vi "Test-Elevator.vi"() -> ()   [LabVIEW 2023]
doc: "This VI implements the framework and scheduler for your robotics program. It should not be necessary to modify the framework. You are expected to add your code to the VIs called from Robot Main - the ones located in the Team Code folder within the project."
uses:
  <vilib>/Rock Robotics/WPI/DriverStation/WPI_DriverStationRobotMode2.ctl
  Robot Global Data.vi
  Elevator/ElevatorL4SendCmd.vi
  Elevator/ElevatorAlgae1SendCmd.vi
  Elevator/ElevatorL3SendCmd.vi
  Elevator/ElevatorAlgae2SendCmd.vi
  Elevator/ElevatorSourceSendCmd.vi
  Elevator/ElevatorL2SendCmd.vi
  Elevator/ElevatorRestSendCmd.vi
  Elevator/ElevatorL1SendCmd.vi
  Elevator/ElevatorGlobal.vi
  <vilib>/Rock Robotics/WPI/ThirdParty/JAS_Junk/TrajLib/Trajectory_Library.lvlib
panel:
  out "Battery_Volts":dbl format="%9.1f"
  out "L4 2":bool
  out "HeightSP_Inch":dbl format="%9.1f"
  in  "Rest":bool
  out "HighLimitSwitch":bool
  in  "CmdSpecific":bool
  in  "Specific":dbl
  in  "Algae2":bool
  in  "L4":bool
  in  "Source":bool
  out "Low Limit Switch":bool
  out "HeightInch":dbl format="%9.1f"
  in  "L1":bool
  in  "L2":bool
  in  "Algae1":bool
  in  "L3":bool
  out "Robot Mode":T1
  out "MotorOutDmd":dbl format="%9.2f"
  in  "error in (no error)":errorcluster
  in  "Finish":bool
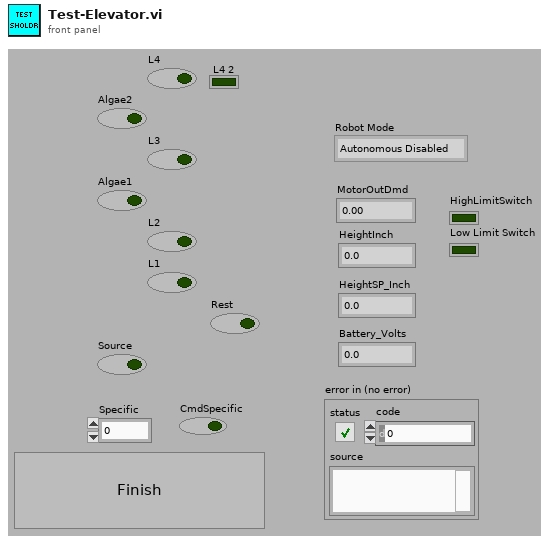
[diagram p1: front panel]
types:
  T1 = typedef "WPI_DriverStationRobotMode2.ctl" = enum16{"Autonomous Disabled", "Autonomous Enabled", "Teleop Disabled", "Teleop Enabled", "Disconnected", "Finish", "Test Disabled", "Test Enabled", "Emergency Stopped"}
  T2 = typedef "WPI_DriverStationMatch Info.ctl" = cluster{"Autonomous Elapsed Seconds":dbl, "TeleOp Elapsed Seconds":dbl, "Disabled Elapsed Seconds":dbl, "Visited Autonomous":bool, "Visited TeleOp":bool, "Visited Disabled":bool, "Autonomous Settings":cluster{"Autonomous Style":enum16{"Iterative", "Independent"}, "VI Refnum":refnum<vi>}}
  T3 = typedef "WPI_DriverStationDerivedRobotMode.ctl" = enum16{"Init", "Execute", "Stop"}
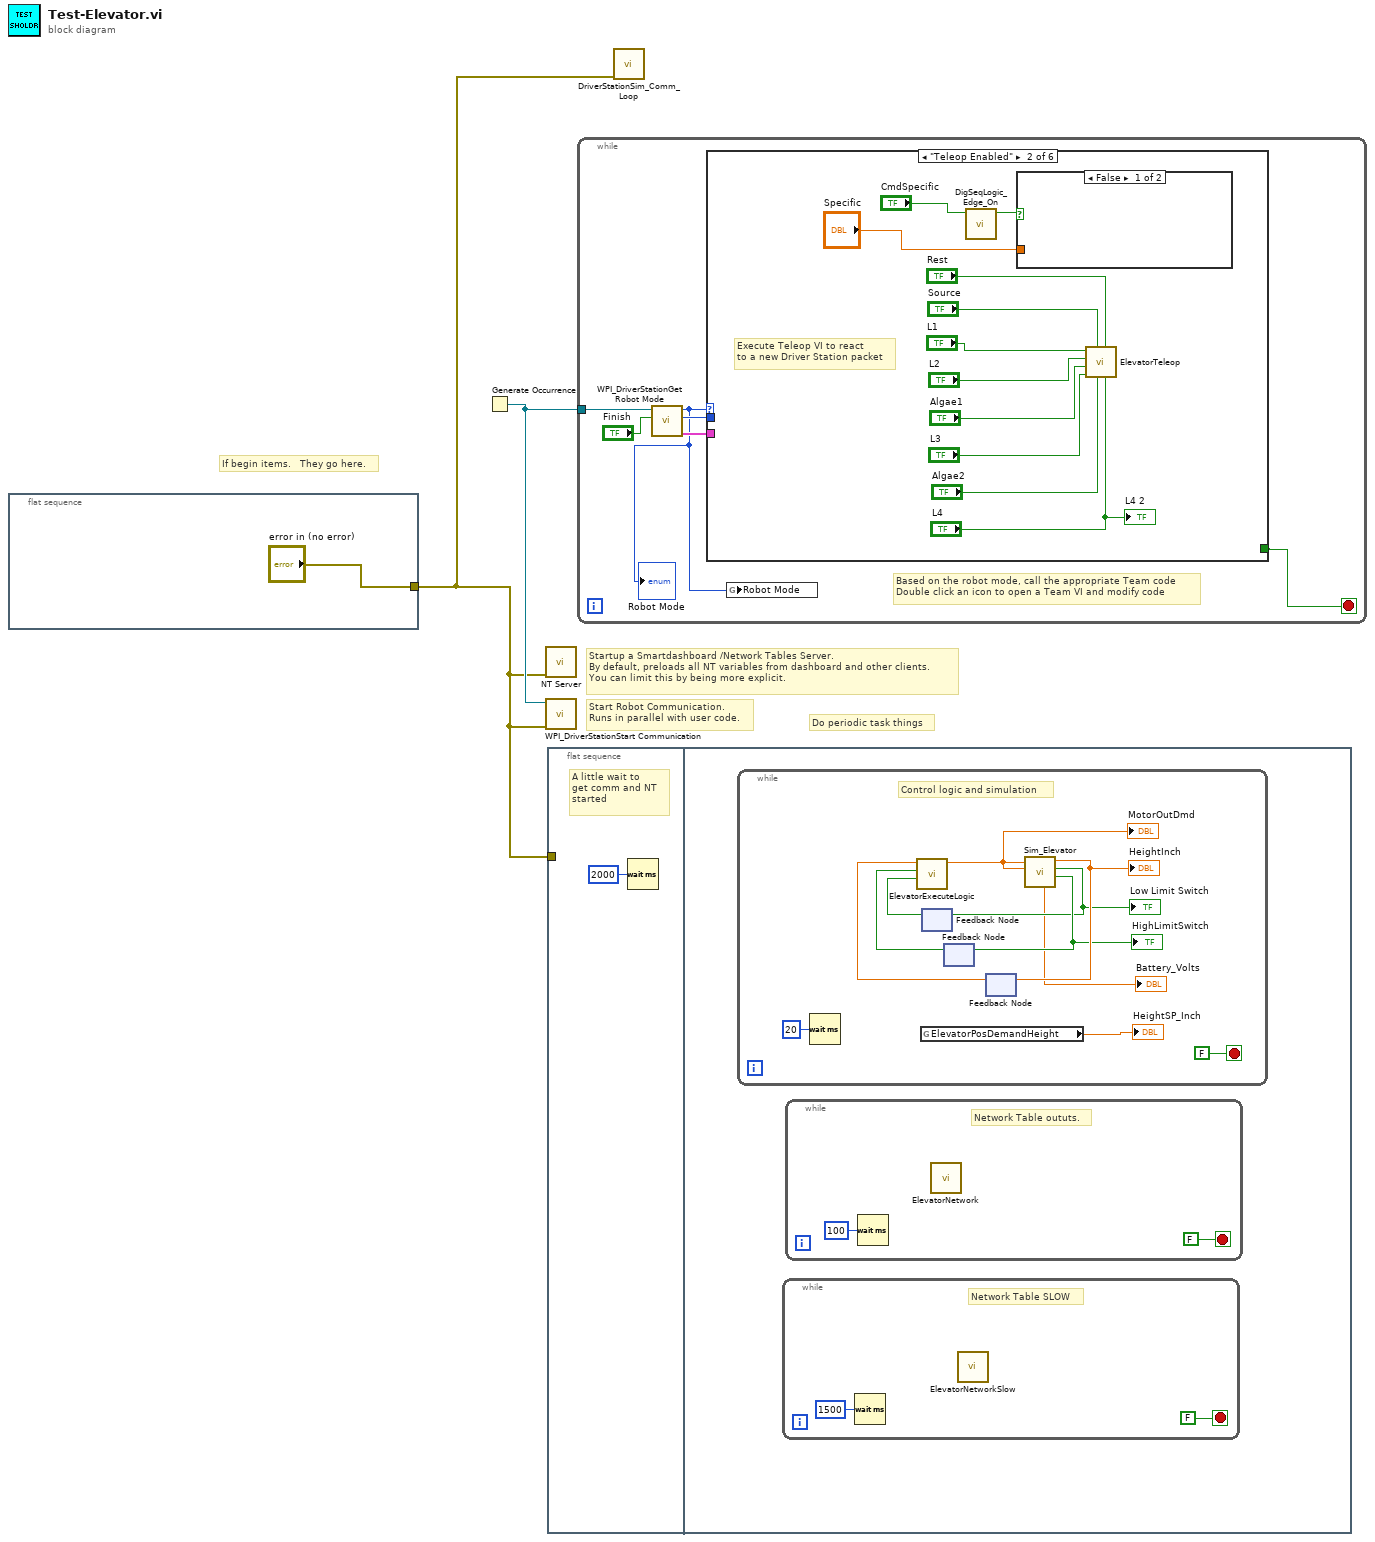
[diagram p0: block diagram]
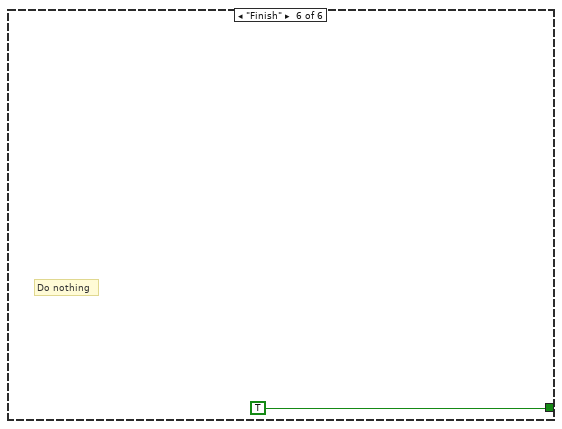
[diagram p7: hidden frame]
diagram:
  # "If begin items.   They go here."
  # "Do periodic task things"
  # "Startup a Smartdashboard /Network Tables Server.\nBy default, preloads all NT variables from dashboard and other clients.\nYou can limit this by being more explicit."
  # "Start Robot Communication.\nRuns in parallel with user code."
  n1 = flat-sequence {
    tunnel: ["error in (no error)"] -> w1
    frame #0 {
    }
  }
  n2 = Generate Occurrence() -> (w2:refnum<k4>)
  n3 = call <vilib>:"NT Server.vi"("error in (no error)"=w1) -> ()  [unwired: 10 in, 1 out]
  n4 = call <vilib>:"WPI_DriverStationStart Communication.vi"("error in (no error)"=w1, "occurrence"=w2) -> ()  [unwired: 1 in, 9 out]
  n5 = flat-sequence {
    tunnel: w1 -> [_]
    frame #0 {
      # "A little wait to\nget comm and NT\nstarted"
      n6 = Wait (ms)(milliseconds to wait=u32 2000) -> ()  [unwired: 1 out]
    }
    frame #1 {
      n7 = while {
        stop <- FALSE stop-if-true
        # "Control logic and simulation"
        n8 = Wait (ms)(milliseconds to wait=u32 20) -> ()  [unwired: 1 out]
        n9 = global read "ElevatorGlobal.vi" "ElevatorPosDemandHeight"() -> (→"HeightSP_Inch":dbl)
        n10 = feedback #1() -> (w13:bool)  [unwired: 1 in]
        n11 = feedback #2() -> (w15:bool)  [unwired: 1 in]
        n12 = feedback #3() -> (w17:dbl)  [unwired: 1 in]
        n13 = call "ElevatorExecuteLogic.vi"("LowLimitSwitch"=w13, "HighLimitSwitch"=w15, "PositionHeight"=w17) -> ("MotorDemand"=w12:dbl)  [unwired: 7 in, 1 out]
        "MotorOutDmd" <- w12
        n14 = call "Sim_Elevator.vi"("Motor2 Dmd"=w12, "Motor1 Dmd"=w12) -> ("HighLimitSwitch"=w16:bool, "Low Limit Switch"=w14:bool, "ElevHeightInch"=w18:dbl, "Voltage"=→"Battery_Volts":dbl)  [unwired: 6 in]
        "HeightInch" <- w18
        "Low Limit Switch" <- w14
        "HighLimitSwitch" <- w16
        n15 = feedback-in #1(w14) -> ()
        n16 = feedback-in #2(w16) -> ()
        n17 = feedback-in #3(w18) -> ()
      }
      n18 = while {
        stop <- FALSE stop-if-true
        # "Network Table SLOW"
        n19 = Wait (ms)(milliseconds to wait=u32 1500) -> ()  [unwired: 1 out]
        n20 = call "ElevatorNetworkSlow.vi"() -> ()  [unwired: 11 in, 1 out]
      }
      n21 = while {
        stop <- FALSE stop-if-true
        # "Network Table oututs."
        n22 = Wait (ms)(milliseconds to wait=u32 100) -> ()  [unwired: 1 out]
        n23 = call "ElevatorNetwork.vi"() -> ()  [unwired: 11 in, 1 out]
      }
    }
  }
  n24 = while {
    tunnel: w2 -> [w25]
    stop <- w20 stop-if-true
    # "Based on the robot mode, call the appropriate Team code\nDouble click an icon to open a Team VI and modify code"
    n25 = call <vilib>:"WPI_DriverStationGet Robot Mode.vi"("Finish"="Finish", "DS Occurrence"=w25) -> ("Match Info out"=w22:T2, "Call Context"=w24:T3, "Robot Mode"=w21:T1)  [unwired: 7 out]
    "Robot Mode" <- w21
    n26 = case shown="\"Teleop Enabled\"" w21 {
      tunnel: w24 -> [_ _ _ _ _ _]
      tunnel: w22 -> [_ _ _ _ _ _]
      tunnel: [_ _ _ _ _ TRUE] -> w20
      frame "Autonomous Enabled" {
        # "Do nothing...."
      }
      frame "Teleop Enabled" {
        # "Execute Teleop VI to react\nto a new Driver Station packet"
        n27 = call <vilib>:"DigSeqLogic_Edge_On.vi"("Input"="CmdSpecific") -> ("On Edge"=w36:bool)  [unwired: 10 in]
        n28 = case shown="False" w36 {
          tunnel: "Specific" -> [_ _]
          frame False {
          }
          frame True {
          }
        }
        n29 = call "ElevatorTeleop.vi"("CmdElevL4"="L4", "CmdElevRest"="Rest", "CmdElevAlgae2"="Algae2", "CmdElevSource"="Source", "CmdElevL3"="L3", "CmdElevAlgae1"="Algae1", "CmdElevL2"="L2", "CmdElevL1"="L1") -> ()  [unwired: 4 in]
        "L4 2" <- "L4"
      }
      frame "Test Disabled", "Test Enabled" {
        # "Do nothing"
      }
      frame "Autonomous Disabled", "Teleop Disabled" {
        # "Do nothing."
      }
      frame "Disconnected", Default {
        # "Driver Station packet didn't arrive.\nPossibly useful for diagnostics"
      }
      frame "Finish" {
        # "Do nothing"
      }
    }
    n30 = global write "Robot Global Data.vi" "Robot Mode"(w21) -> ()
  }
  n31 = call <vilib>:"DriverStationSim_Comm_Loop.vi"("error in (no error)"=w1) -> ()  [unwired: 11 in]
